vi "CreatePizza.vi"(8 "error in (no error)":errorcluster, 11 "PizzaStore in":refnum<class "PizzaStore.lvclass">) -> (0 "error out":errorcluster, 2 "Pizza":string, 3 "PizzaStore out":refnum<class "PizzaStore.lvclass">)   [LabVIEW 2013, in "PizzaStore.lvclass"]
uses:
  PizzaStore.lvclass
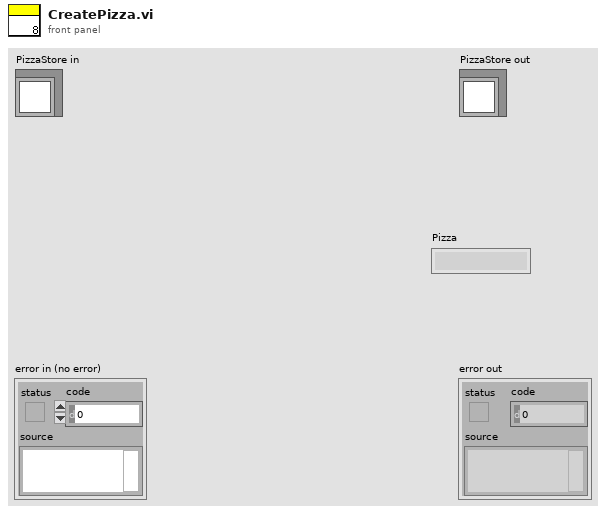
[diagram p1: front panel]
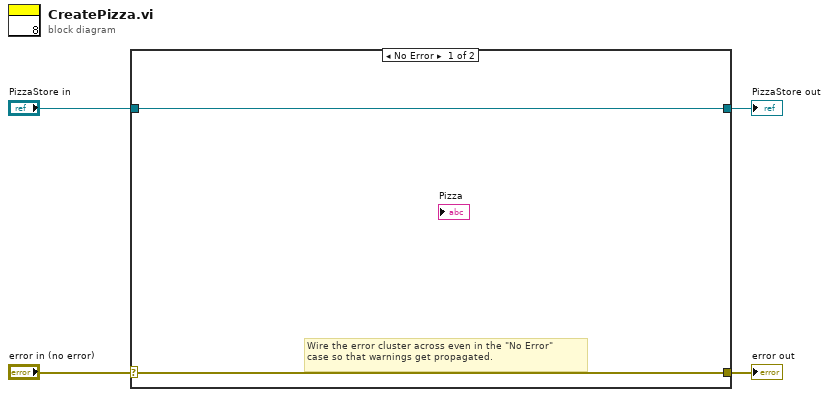
[diagram p0: block diagram]
diagram:
  n1 = case shown="No Error" "error in (no error)" {
    selector: "error in (no error)" -> [w5 w8]
    tunnel: [w5 w8] -> w3
    tunnel: [w6 w7] -> w1
    tunnel: "PizzaStore in" -> [w6 w7]
    frame No Error {
      # "Wire the error cluster across even in the \"No Error\"\ncase so that warnings get propagated."
    }
    frame Error {
    }
  }
  "error out" <- w3
  "PizzaStore out" <- w1
